vi "AlliGator Fit Phasor Ratio Plot v2.vi"(8 "Error In":errorcluster, 10 "Mouse Coordinates":T1, 11 "Phasor Ratio Graph Ref":refnum<vi>) -> (0 "Error Out":errorcluster, 1 "Message":string, 2 "Intercept":dbl, 3 "Slope":dbl)   [LabVIEW 2021, in "AlliGator Phasor Ratio.lvlib"]
doc: "Fits phasor ratio plot to a line."
uses:
  AlliGator Phasor Ratio.lvlib
  <vilib>/Utility/miscctls.llb/LVPoint32TypeDef.ctl
  <vilib>/Analysis/6fits.llb/Curve Fitting Criteria.ctl
  Graphs/LabVIEW Plot Interpolation.ctl
  Graphs/Get Plot at Mouse Click (XY Graph)/Get Plot at Mouse Click [AAC].vi
  Graphs/XY Graph/XY Graph Add Single Plot with Name.vi
  <vilib>/Analysis/NI_AALPro.lvlib
  Graphs/XY Graph/XY Graph Add-Ons.lvlib
  Graphs/Graphs.lvlib
  Error/Error.lvlib
  Math/Math.lvlib
panel:
  # "see the AlliGator License on the block diagram (Ctrl+E or Window:Show Block Diagram)"
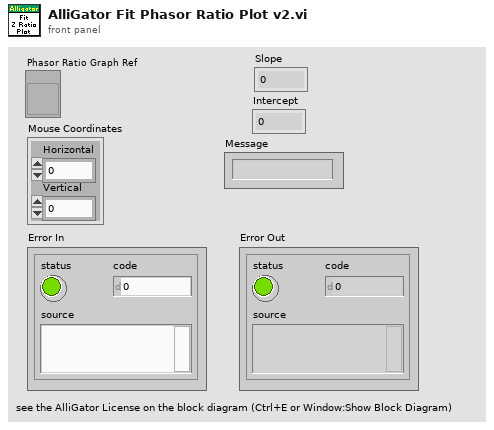
[diagram p1: front panel]
types:
  T1 = typedef "LVPoint32TypeDef.ctl" = cluster{"Horizontal":i32, "Vertical":i32}
  T2 = typedef "XY Graph Add-Ons.lvlib/XY Graph Refnum.ctl" = refnum<vi>
  T3 = typedef "NI_AALPro.lvlib/Curve Fitting Criteria.ctl" = u16
  T4 = typedef "Graphs.lvlib/LabVIEW Plot Interpolation.ctl" = u8
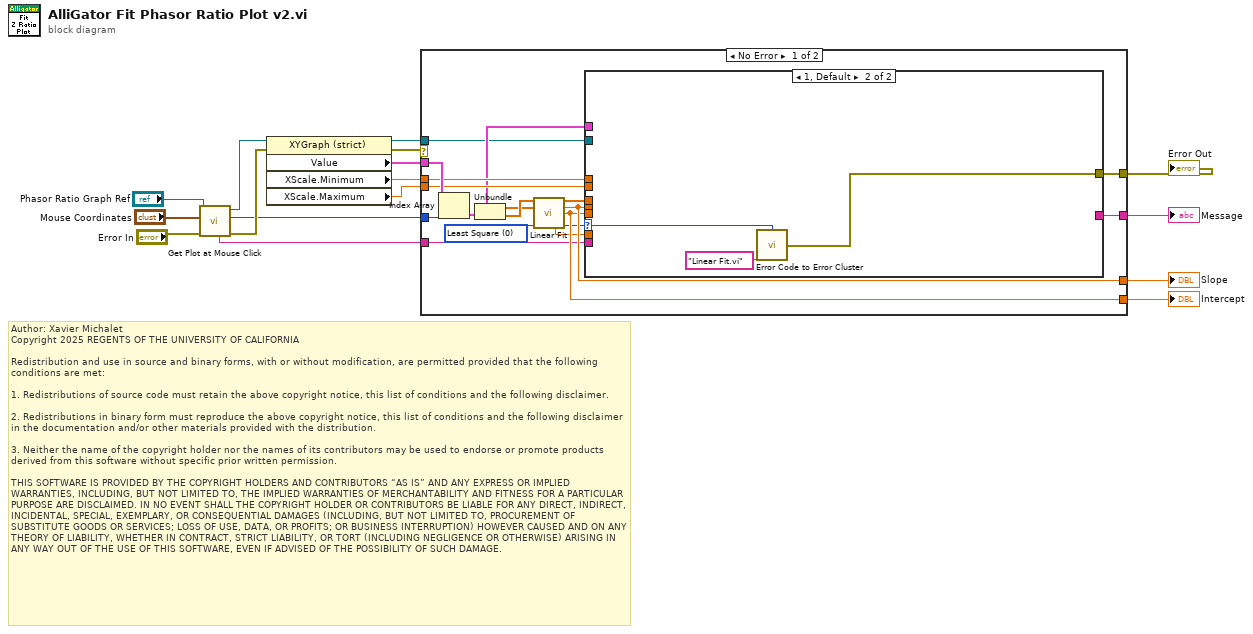
[diagram p0: block diagram]
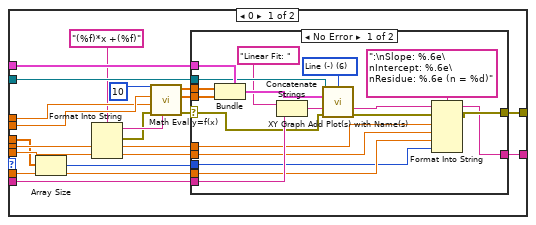
[diagram p2: hidden frame]
diagram:
  # "Author: Xavier Michalet\nCopyright 2025 REGENTS OF THE UNIVERSITY OF CALIFORNIA\n\nRedistribution and use in source and binary forms, with or without modification, are permitted provided that the following conditions are met:\n\n1. Redistributions of source code must retain the above copyright notice, this list of conditions and the following disclaimer.\n\n2. Redistributions in binary form must reproduce the above copyright notice, this list of conditions and the following disclaimer in the documentation and/or other materials provided with the distribution.\n\n3. Neither the name of the copyright holder nor the names of its contributors may be used to endorse or promote products derived from this software without specific prior written permission.\n\nTHIS SOFTWARE IS PROVIDED BY THE COPYRIGHT HOLDERS AND CONTRIBUTORS “AS IS” AND ANY EXPRESS OR IMPLIED WARRANTIES, INCLUDING, BUT NOT LIMITED TO, THE IMPLIED WARRANTIES OF MERCHANTABILITY AND FITNESS FOR A PARTICULAR PURPOSE ARE DISCLAIMED. IN NO EVENT SHALL THE COPYRIGHT HOLDER OR CONTRIBUTORS BE LIABLE FOR ANY DIRECT, INDIRECT, INCIDENTAL, SPECIAL, EXEMPLARY, OR CONSEQUENTIAL DAMAGES (INCLUDING, BUT NOT LIMITED TO, PROCUREMENT OF SUBSTITUTE GOODS OR SERVICES; LOSS OF USE, DATA, OR PROFITS; OR BUSINESS INTERRUPTION) HOWEVER CAUSED AND ON ANY THEORY OF LIABILITY, WHETHER IN CONTRACT, STRICT LIABILITY, OR TORT (INCLUDING NEGLIGENCE OR OTHERWISE) ARISING IN ANY WAY OUT OF THE USE OF THIS SOFTWARE, EVEN IF ADVISED OF THE POSSIBILITY OF SUCH DAMAGE."
  n1 = call-poly "Get Plot at Mouse Click.vi"("error in (no error)"="Error In", "Mouse Click Coordinates"="Mouse Coordinates", "XYGraph Ref"="Phasor Ratio Graph Ref") -> ("error out"=w7:errorcluster, "Plot at Coordinates"=w6:i32, "XYGraph Ref"=w8:T2, "Plot Name"=w3:string)  [unwired: 2 in, 3 out]
  n2 = property class="XYGraph (strict)"(reference=w8, error in=w7) -> (reference out=w5:T2, error out=w4:errorcluster, "Value"=w16:cluster{"X Array":dbl[], "Y Array":dbl[]}[], "XScale.Minimum"=w15:dbl, "XScale.Maximum"=w14:dbl)
  n3 = case shown="No Error" w4 {
    selector: w4 -> [_ w76]
    tunnel: w16 -> [w33 _]
    tunnel: w15 -> [w31 _]
    tunnel: w14 -> [w30 _]
    tunnel: [w29 _] -> w13
    tunnel: [w28 _] -> w12
    tunnel: w6 -> [w26 _]
    tunnel: w5 -> [w23 _]
    tunnel: [w22 w76] -> w1
    tunnel: w3 -> [w20 _]
    tunnel: [w19 _] -> w2
    frame No Error {
      w32 = T3 0 items=["Least Square", "Least Absolute Residual", "Bisquare"] ("method")
      n4 = Index Array(array=w33, index=w26) -> (element=w27:cluster{"X Array":dbl[], "Y Array":dbl[]})
      n5 = Unbundle(w27) -> ("X Array"=w24:dbl[], "Y Array"=w25:dbl[])
      n6 = call <vilib>:"Linear Fit.vi"("Y"=w25, "X"=w24, "method"=w32) -> ("Best Linear Fit"=w17:dbl[], "slope"=w29:dbl, "intercept"=w28:dbl, "residue"=w18:dbl, "error"=w21:i32)  [unwired: 8 in]
      n7 = case shown="1, Default" w21 {
        selector: w21 -> [_ w75]
        tunnel: w31 -> [w40 _]
        tunnel: w30 -> [w41 _]
        tunnel: w29 -> [w47 _]
        tunnel: w28 -> [w46 _]
        tunnel: w27 -> [w52 _]
        tunnel: w23 -> [w51 _]
        tunnel: [w50 w74] -> w22
        tunnel: w20 -> [w49 _]
        tunnel: [w48 _] -> w19
        tunnel: w18 -> [w45 _]
        tunnel: w17 -> [w44 _]
        frame 0 {
          n8 = Array Size(array=w44) -> (size(s)=w43:i32)
          n9 = Format Into String(format string="(%f)*x +(%f)", w47, w46) -> (resulting string=w35:string, error out=w34:errorcluster)  [unwired: 2 in]
          n10 = call "Math Eval y=f(x).vi"("formula"=w35, "Error In"=w34, "start"=w40, "end"=w41, "number of points"=u32 10) -> ("Error Out"=w39:errorcluster, "Y Values"=w37:dbl[], "X Values"=w38:dbl[])  [unwired: 3 in, 1 out]
          n11 = case shown="No Error" w39 {
            selector: w39 -> [w53 w72]
            tunnel: w52 -> [w71 _]
            tunnel: w51 -> [w69 _]
            tunnel: [w64 w72] -> w50
            tunnel: w49 -> [w68 _]
            tunnel: [w63 _] -> w48
            tunnel: w47 -> [w62 _]
            tunnel: w46 -> [w61 _]
            tunnel: w45 -> [w59 _]
            tunnel: w43 -> [w58 _]
            tunnel: w38 -> [w55 _]
            tunnel: w37 -> [w54 _]
            frame No Error {
              w57 = T4 6 items=["Point (.)", "Stepwise Right (--.)", "Line + Point (\\. /)", "Stepwise Left (.--)", "Stepwise Centered (-.-)", "Stepwise Vertical (|.|)", "Line (-)", "Use Previous Plot's Style"] ("Plot Interpolation (Previous Plot's Style)")
              n12 = Bundle(cluster=w71, "X Array"=w55, "Y Array"=w54) -> (w70:cluster{"X Array":dbl[], "Y Array":dbl[]})
              n13 = Concatenate Strings("Linear Fit: " ("string"), w68) -> (w66:string)
              n14 = call-poly "XY Graph Add Plot(s) with Name(s).vi"("XYGraph Ref in"=w69, "Plot Interpolation (Previous Plot's Style)"=w57, "Plot"=w70, "Plot Name (\"Plot\")"=w66, "error in (no error)"=w53) -> ("Plot Name"=w65:string, "error out"=w56:errorcluster)  [unwired: 7 in, 2 out]
              n15 = Format Into String(format string=":\nSlope: %.6e\nIntercept: %.6e\nResidue: %.6e (n = %d)", initial string=w65, error in=w56, w62, w61, w59, w58) -> (resulting string=w63:string, error out=w64:errorcluster)
            }
            frame Error {
            }
          }
        }
        frame 1, Default {
          n16 = call "Error Code to Error Cluster.vi"("Error Code"=w75, "Error Source"="Linear Fit.vi") -> ("Error Out"=w74:errorcluster)  [unwired: 13 in]
        }
      }
    }
    frame Error {
    }
  }
  "Slope" <- w13
  "Intercept" <- w12
  "Error Out" <- w1
  "Message" <- w2
